vi "Start UI.vi"(8 "error in (no error)":errorcluster, 11 "Client UI in":refnum<class "Client UI.lvclass">) -> (0 "error out":errorcluster, 3 "Client UI out":refnum<class "Client UI.lvclass">)   [LabVIEW 2016, in "Client UI.lvlib" / "Client UI.lvclass"]
uses:
  Client UI.lvclass
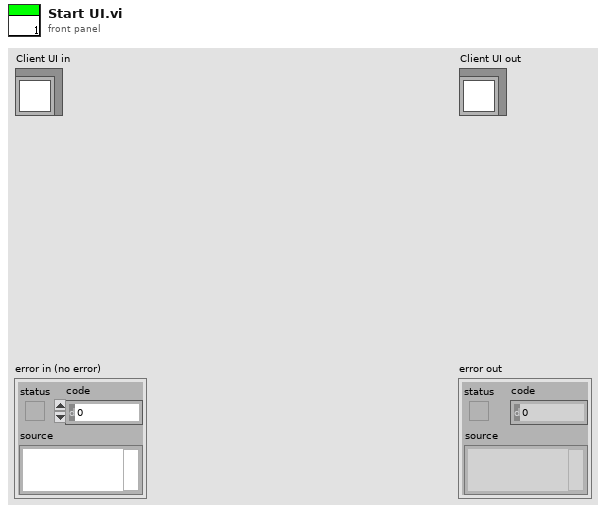
[diagram p1: front panel]
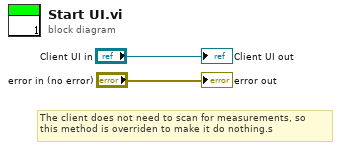
[diagram p0: block diagram]
diagram:
  # "The client does not need to scan for measurements, so \nthis method is overriden to make it do nothing.s"
  "error out" <- "error in (no error)"
  "Client UI out" <- "Client UI in"
